vi "OutputToXML.vi"(8 "error in (no error)":errorcluster, 11 "LSEPlugin in":refnum<class "LSEPlugin.lvclass">) -> (0 "error out":errorcluster, 2 "AppOutputData out":variant)   [LabVIEW 2014, in "AppPlugins.lvlib" / "LSEPlugin.lvclass"]
uses:
  LSEPlugin.lvclass
  Typedefs/LSEOutput.ctl
  Typedefs/LSEConfig.ctl
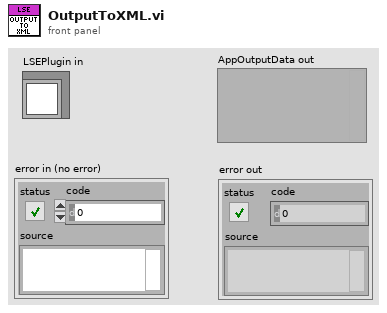
[diagram p1: front panel]
types:
  T1 = typedef "AppPlugins.lvlib/LSEPlugin.lvclass/LSEOutput.ctl" = cluster{"SystemVoltagesRef":cdb[][], "Vestimate":cdb[][], "LSEConfig":T2, "Bus":dbl[]}
  T2 = typedef "AppPlugins.lvlib/LSEPlugin.lvclass/LSEConfig.ctl" = cluster{"NoiseVariance":dbl, "IEEESystem":u32, "PMULocations":u32[], "Vindex":i32, "Iindex":i32, "DynamicRef":string}
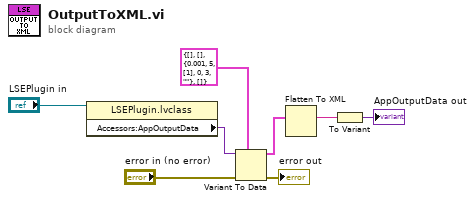
[diagram p0: block diagram]
diagram:
  n1 = property class="LSEPlugin.lvclass"(reference="LSEPlugin in") -> ("Accessors:AppOutputData"=w7:variant)  [unwired: 1 in, 2 out]
  n2 = Variant To Data(error in="error in (no error)", type=T1 {"SystemVoltagesRef"=[], "Vestimate"=[], "LSEConfig"={"NoiseVariance"=0.001, "IEEESystem"=5, "PMULocations"=[1], "Vindex"=0, "Iindex"=3, "DynamicRef"=""}, "Bus"=[]} ("LSEOutput"), Variant=w7) -> (data=w3:T1, error out=→"error out":errorcluster)
  n3 = Flatten To XML(anything=w3) -> (xml string=w2:string)
  n4 = To Variant(anything=w2) -> (Variant=→"AppOutputData out":variant)
